vi "Generate Non Text Layer(s).vi"(0 "Library Path":path, 5 "new picture":picture, 11 "error in":errorcluster) -> (4 "Layers":refnum<class "Layer.lvclass">[](array[class]), 15 "error out":errorcluster)   [LabVIEW 2021, in "Text-Based VI Icon.lvlib"]
uses:
  Text-Based VI Icon.lvlib
  lv_icon/Classes/Layer/Layer.lvclass
  lv_icon/Controls/Layer.ctl
  User Visible Strings.vi
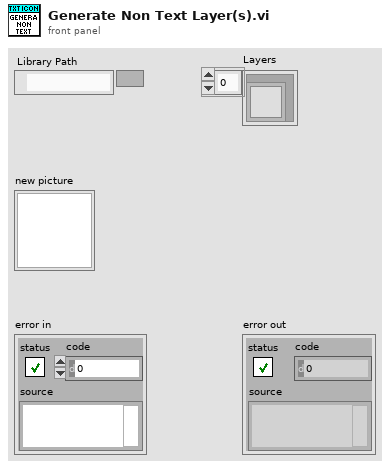
[diagram p1: front panel]
types:
  T1 = cluster{"left":i16, "top":i16, "right":i16, "bottom":i16}
  T2 = typedef "Layer.ctl" = cluster{"LayerIcon":picture, "LayerName":string, "Opacity":u8, "Visibility?":bool}
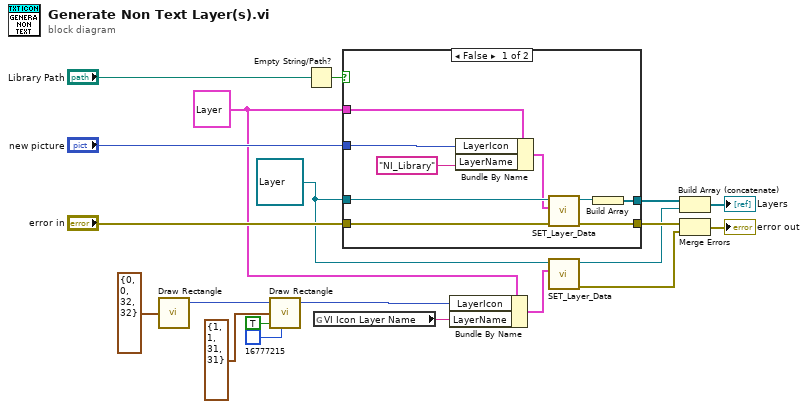
[diagram p0: block diagram]
diagram:
  w1 = T2 {"LayerIcon"=bytes[3102], "LayerName"="", "Opacity"=100, "Visibility?"=TRUE} ("Data")
  w18 = refnum<class "Layer.lvclass"> refnum ("Layer.lvclass in")
  n1 = call <vilib>:"Draw Rectangle.vi"("rect"=T1 {"left"=0, "top"=0, "right"=32, "bottom"=32}) -> ("new picture"=w16:picture)  [unwired: 8 in]
  n2 = call <vilib>:"Draw Rectangle.vi"("picture"=w16, "rect"=T1 {"left"=1, "top"=1, "right"=31, "bottom"=31}, "fill?(F)"=TRUE, "color(black)"=u32 16777215) -> ("new picture"=w14:picture)  [unwired: 5 in]
  n3 = Empty String/Path?(string/path="Library Path") -> (empty?=w19:bool)
  n4 = global read "User Visible Strings.vi" "VI Icon Layer Name"() -> (w10:string)
  n5 = case shown="False" w19 {
    tunnel: "error in" -> [w27 w30]
    tunnel: w18 -> [w29 _]
    tunnel: w1 -> [w28 _]
    tunnel: [w23 w30] -> w9
    tunnel: [w22 _] -> w7
    tunnel: "new picture" -> [w21 _]
    frame False {
      n6 = Bundle By Name(cluster=w28, "LayerIcon"=w21, "LayerName"="NI_Library") -> (w26:T2)
      n7 = call-dynamic "SET_Layer_Data.vi"("error in (no error)"=w27, "Data"=w26, "Layer.lvclass in"=w29) -> ("error out"=w23:errorcluster, "Layer.lvclass out"=w24:refnum<class "Layer.lvclass">)  [unwired: 7 in]
      n8 = Build Array(w24) -> (w22:refnum<class "Layer.lvclass">[])
    }
    frame True {
    }
  }
  n9 = Bundle By Name(cluster=w1, "LayerIcon"=w14, "LayerName"=w10) -> (w11:T2)
  n10 = call-dynamic "SET_Layer_Data.vi"("Data"=w11, "Layer.lvclass in"=w18) -> ("error out"=w8:errorcluster, "Layer.lvclass out"=w6:refnum<class "Layer.lvclass">)  [unwired: 8 in]
  n11 = Build Array (concatenate)(w7, w6) -> (→"Layers":refnum<class "Layer.lvclass">[])
  n12 = Merge Errors(w9, w8) -> (→"error out":errorcluster)
